vi "RuleConvert.vi"(8 "Error In":errorcluster, 11 "String":string) -> (0 "Error Out":errorcluster, 2 "Dead rule":i32[](array[numeric]), 3 "Live rule":i32[](array[numeric]))   [LabVIEW 2020]
doc: "Convert string \"xxx/yyy\" which describie rule of live and dead to arrays of numbers to compare."
uses:
  <userlib>/_OpenG.lib/array/array.llb/Remove Duplicates from 1D Array (I32)__ogtk.vi
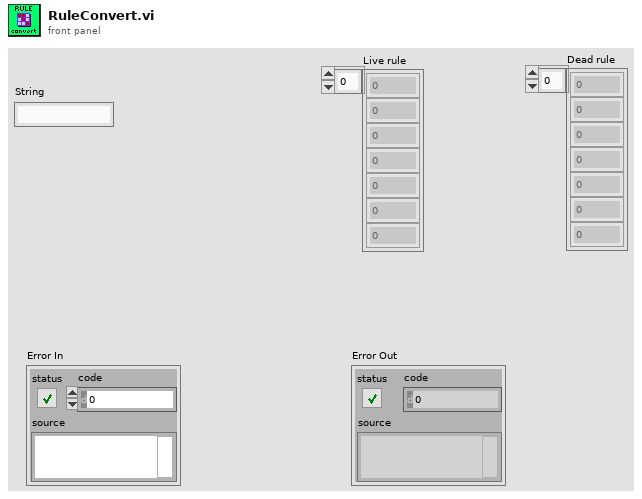
[diagram p1: front panel]
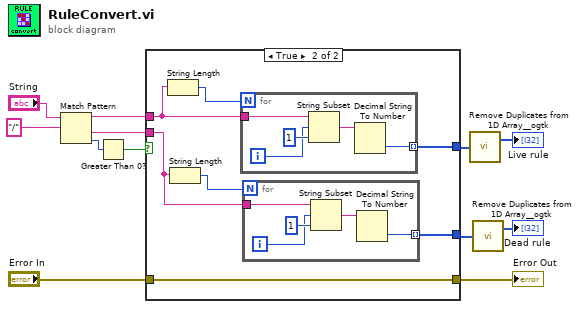
[diagram p0: block diagram]
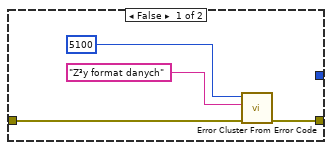
[diagram p2: hidden frame]
diagram:
  n1 = Match Pattern(string="String", regular expression="/") -> (before substring=w9:string, after substring=w10:string, offset past match=w8:i32)  [unwired: 1 in, 1 out]
  n2 = Greater Than 0?(x=w8) -> (x > 0?=w7:bool)
  n3 = case shown="True" w7 {
    tunnel: w10 -> [_ w19]
    tunnel: w9 -> [_ w23]
    tunnel: [_ w21] -> w6
    tunnel: [_ w18] -> w4
    tunnel: "Error In" -> [w16 w17]
    tunnel: [w15 w17] -> w1
    frame False {
      n4 = call <vilib>:"Error Cluster From Error Code.vi"("error in (no error)"=w16, "error message (\"\")"="Z³y format danych" ("error message (\"\")"), "error code (0)"=5100) -> ("error out"=w15:errorcluster)  [unwired: 6 in]
    }
    frame True {
      n5 = String Length(string=w23) -> (length=w22:i32)
      n6 = String Length(string=w19) -> (length=w20:i32)
      n7 = for {
        N: w22 -> [_]
        tunnel: w23 -> [w33]
        tunnel: [w29] -> w21 mode=indexing
        i -> [w31]
        n8 = String Subset(string=w33, offset (0)=w31, length (rest)=1 ("length (rest)")) -> (substring=w30:string)
        n9 = Decimal String To Number(string=w30) -> (number=w29:i32)  [unwired: 2 in, 1 out]
      }
      n10 = for {
        N: w20 -> [_]
        tunnel: w19 -> [w28]
        tunnel: [w24] -> w18 mode=indexing
        i -> [w26]
        n11 = String Subset(string=w28, offset (0)=w26, length (rest)=1 ("length (rest)")) -> (substring=w25:string)
        n12 = Decimal String To Number(string=w25) -> (number=w24:i32)  [unwired: 2 in, 1 out]
      }
    }
  }
  "Error Out" <- w1
  n13 = call-poly <userlib>:"Remove Duplicates from 1D Array__ogtk.vi"("Input Array"=w6) -> ("Output Array"=→"Live rule":i32[])  [unwired: 1 out]
  n14 = call-poly <userlib>:"Remove Duplicates from 1D Array__ogtk.vi"("Input Array"=w4) -> ("Output Array"=→"Dead rule":i32[])  [unwired: 1 out]
